vi "Generate Action Event.vi"(8 "error in (no error)":errorcluster, 9 "Description":string, 10 "Action":T1, 11 "Artifactory in":refnum<class "Artifactory.lvclass">) -> (0 "error out":errorcluster, 3 "Artifactory out":refnum<class "Artifactory.lvclass">)   [LabVIEW 2021, in "Artifactory.lvclass"]
uses:
  Artifactory.lvclass
  Actions -- enum.ctl
  Repository Event -- cluster.ctl
  Artifactory.lvclass/Artifactory.ctl
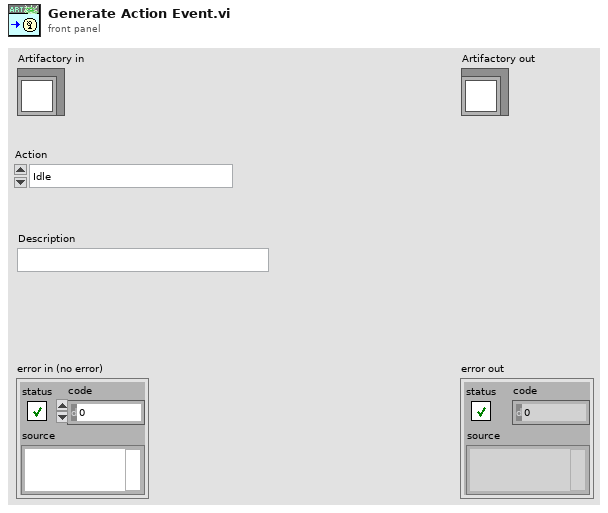
[diagram p1: front panel]
types:
  T1 = typedef "Artifactory.lvclass/Actions -- enum.ctl" = enum16{"Idle", "Custom Event", "Connecting to Artifactory", "Verifying Permissions", "Listing local repository", "Listing remote repository", "Computing changes", "Uploading file", "Downloading file"}
  T2 = typedef "Artifactory.lvclass/Repository Event -- cluster.ctl" = cluster{"Action":T1, "Description":string}
  T3 = typedef "Artifactory.lvclass/Public Events -- cluster.ctl" = cluster{"Action":refnum<user-event>}
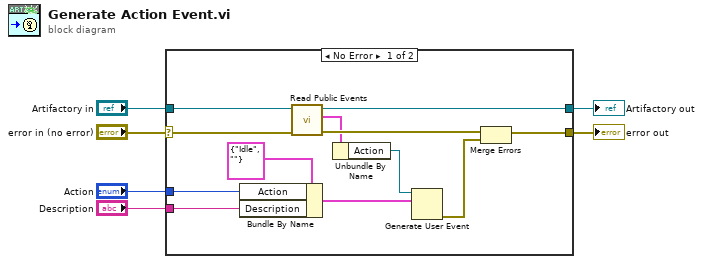
[diagram p0: block diagram]
diagram:
  n1 = case shown="No Error" "error in (no error)" {
    selector: "error in (no error)" -> [w10 w20]
    tunnel: [w13 w20] -> w5
    tunnel: [w12 w19] -> w3
    tunnel: "Artifactory in" -> [w11 w19]
    tunnel: "Action" -> [w17 _]
    tunnel: "Description" -> [w16 _]
    frame No Error {
      n2 = Bundle By Name(cluster=T2 {"Action"=enum."Idle", "Description"=""} ("Event"), "Action"=w17, "Description"=w16) -> (w15:T2)
      n3 = call-dynamic "Read Public Events.vi"("error in (no error)"=w10, "Artifactory in"=w11) -> ("error out"=w9:errorcluster, "Public Events"=w8:T3, "Artifactory out"=w12:refnum<class "Artifactory.lvclass">)  [unwired: 7 in]
      n4 = Unbundle By Name(w8) -> ("Action"=w7:refnum<user-event>)
      n5 = Generate User Event(user event=w7, event data cluster=w15) -> (error out=w14:errorcluster)  [unwired: 2 in, 1 out]
      n6 = Merge Errors(w9, w14) -> (w13:errorcluster)
    }
    frame Error {
    }
  }
  "error out" <- w5
  "Artifactory out" <- w3
